vi "Obtain Priority Queue.vi"(8 "error in (no error)":errorcluster) -> (0 "error out":errorcluster, 3 "Priority Message Queue out":refnum<class "Priority Message Queue.lvclass">)   [LabVIEW 2020, in "Artifex.lvlib" / "Priority Message Queue.lvclass"]
uses:
  Priority Message Queue.lvclass
  Message/Message.lvclass
  Ref Data.ctl
  Priority.ctl
  Artifex.lvlib
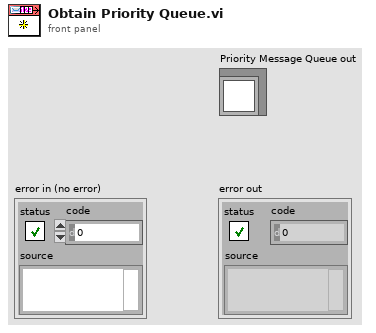
[diagram p1: front panel]
types:
  T1 = typedef "Artifex.lvlib/Priority.ctl" = enum16{"Low", "Normal", "High"}
  T2 = typedef "Artifex.lvlib/Priority Message Queue.lvclass/Ref Data.ctl" = cluster{"# Waiting":u32, "Buffers":refnum<queue>[], "Wait Msg":refnum<queue>, "Wait Prior":refnum<queue>}
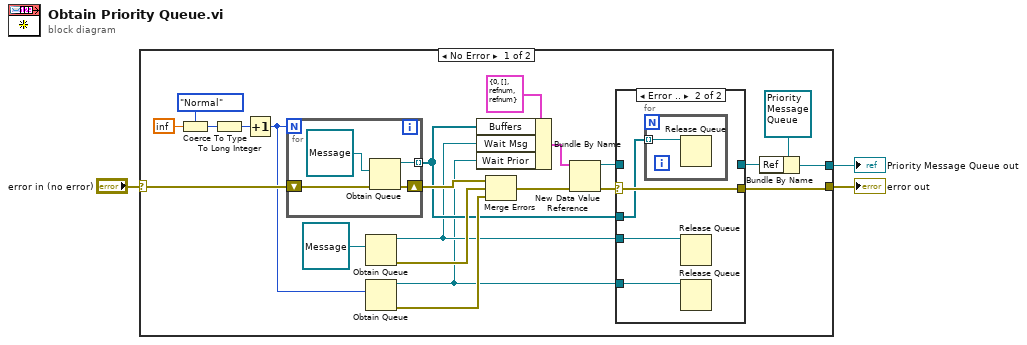
[diagram p0: block diagram]
diagram:
  n1 = case shown="No Error" "error in (no error)" {
    selector: "error in (no error)" -> [w22 w37]
    tunnel: [w10 _] -> w3
    tunnel: [w9 w37] -> w1
    frame No Error {
      n2 = Coerce To Type(0:inf, 1:Priority."Normal" ("Priority")) -> (2:w6:T1)
      n3 = To Long Integer(number=w6) -> (32bit integer=w5:i32)
      n4 = Increment(x=w5) -> (x+1=w8:i32)
      n5 = for {
        N: w8 -> [_]
        shift-right: [w35] -> w25
        shift-left: w22 -> [w36]
        tunnel: [w33] -> w15 mode=indexing
        n6 = Obtain Queue(element data type=refnum<class "Message.lvclass"> refnum ("Artifex.lvlib:Message.lvclass"), error in (no error)=w36) -> (queue out=w33:refnum<queue>, error out=w35:errorcluster)  [unwired: 3 in, 1 out]
      }
      n7 = Obtain Queue(element data type=refnum<class "Message.lvclass"> refnum ("Artifex.lvlib:Message.lvclass")) -> (queue out=w14:refnum<queue>, error out=w24:errorcluster)  [unwired: 4 in, 1 out]
      n8 = Obtain Queue(element data type=w8) -> (queue out=w13:refnum<queue>, error out=w23:errorcluster)  [unwired: 4 in, 1 out]
      n9 = Bundle By Name(cluster=T2 {"# Waiting"=0, "Buffers"=[], "Wait Msg"=refnum, "Wait Prior"=refnum} ("Priority Queue Internals"), "Buffers"=w15, "Wait Msg"=w14, "Wait Prior"=w13) -> (w18:T2)
      n10 = Merge Errors(w25, w24, w23) -> (w19:errorcluster)
      n11 = New Data Value Reference(data value=w18, error in=w19) -> (data value reference=w16:refnum<data-value>, error out=w17:errorcluster)
      n12 = case shown="Error .." w17 {
        selector: w17 -> [w26 w31]
        tunnel: [w27 _] -> w12
        tunnel: w16 -> [w27 _]
        tunnel: w15 -> [_ w30]
        tunnel: w14 -> [_ w29]
        tunnel: w13 -> [_ w28]
        tunnel: [w26 w31] -> w9
        frame No Error {
        }
        frame Error {
          n13 = for {
            tunnel: w30 -> [w32] mode=indexing
            n14 = Release Queue(queue=w32) -> ()  [unwired: 2 in, 3 out]
          }
          n15 = Release Queue(queue=w29) -> ()  [unwired: 2 in, 3 out]
          n16 = Release Queue(queue=w28) -> ()  [unwired: 2 in, 3 out]
        }
      }
      n17 = Bundle By Name(cluster=refnum<class "Priority Message Queue.lvclass"> refnum ("Priority Message Queue in"), "Ref"=w12) -> (w10:refnum<class "Priority Message Queue.lvclass">)
    }
    frame Error {
    }
  }
  "error out" <- w1
  "Priority Message Queue out" <- w3
